vi "RetrieveCustomDiagPacket.vi"(8 "error in":errorcluster, 10 "statusItems":T1[](array[typedef]) {"item code" items=["AccelerationCommand"=6, "AccelerationCommandDrive"=181, "AccelerationCommandRaw"=50, "AccelerationCommandRawCal"=193, "AccelerationError"=223, "AccelerationFeedback"=192, "AccelerationMode"=144, "AccelerationRate"=140, "AccelerationTime"=138, "AccelerationType"=142, "AccuracyCorrectionEndingPosition"=418, "AccuracyCorrectionStartingPosition"=417, "AnalogInput0"=10, "AnalogInput1"=11, "AnalogInput2"=28, "AnalogInput3"=29, "AnalogOutput0"=36, "AnalogOutput1"=37, "AnalogOutput2"=38, "AnalogOutput3"=39, "AutoFocusError"=410, "AxisFault"=49, "AxisParameter"=76, "AxisStatus"=48, "Backlash"=81, "BacklashTarget"=196, "CalibrationAdjustmentState"=416, "CalibrationAdjustmentValue"=200, "CommunicationRealTimeErrors"=93, "CoordinatedDistanceRemaining"=272, "CoordinatedPositionTarget"=46, "CurrentCommand"=8, "CurrentError"=9, "CurrentFeedback"=7, "CurrentFeedbackAverage"=73, "DecelerationMode"=145, "DecelerationRate"=141, "DecelerationTime"=139, "DecelerationType"=143, "DigitalInput"=15, "DigitalOutput"=16, "DistanceLog"=378, "DriveAssert"=453, "DriveCommandsDelayed"=424, "DriveCommandsLost"=425, "DriveCommunicationDelay"=253, "DriveCommunicationDelayLive"=254, "DriveInterfaceCommandCode"=191, "DriveInterfacePacketBit"=261, "DriveInterfacePacketDouble"=189, "DriveInterfacePacketFloat"=190, "DriveInterfacePacketInfoBitValue"=210, "DriveInterfacePacketInt16"=187, "DriveInterfacePacketInt32"=186, "DriveInterfacePacketInt8"=188, "DriveInterfacePacketResponseBit"=262, "DriveInterfacePacketResponseDouble"=259, "DriveInterfacePacketResponseFloat"=260, "DriveInterfacePacketResponseInt16"=257, "DriveInterfacePacketResponseInt32"=256, "DriveInterfacePacketResponseInt8"=258, "DriveInterfacePacketStreamingData"=226, "DriveMotionDelay"=199, "DriveMotionDelayLive"=252, "DriveMotionRate"=198, "DriveSMCMotionState"=168, "DriveStatus"=47, "DriveStatusActual"=99, "FeedforwardCurrent"=208, "FixtureOffset"=18, "FreezeVelocityCommand"=238, "FreezeVelocityFeedback"=239, "GainAffScale"=130, "GainKd1Scale"=333, "GainKiScale"=127, "GainKp1Scale"=334, "GainKpiScale"=129, "GainKposScale"=126, "GainKpScale"=128, "GainVffScale"=131, "GalvoLaserOffDelay"=413, "GalvoLaserOnDelay"=412, "GalvoLaserOutputRaw"=183, "GalvoLaserOutputRawAdvance"=411, "GantryMarkerLatchPosition"=368, "GantryOffset"=91, "GantryRealignState"=100, "HomeState"=82, "InternalPositionOffsets"=241, "JerkCommandRaw"=89, "JogTrajectoryStatus"=116, "MoveReferenceCornerOffset"=359, "MoveReferenceCutterOffset"=358, "MoveReferencePosition"=339, "MoveReferenceTotalOffset"=360, "NormalcyDebug"=84, "PeakCurrent"=78, "PiezoVoltageCommand"=376, "PiezoVoltageFeedback"=377, "PingTest"=117, "PositionCalibration2D"=83, "PositionCalibrationAll"=55, "PositionCalibrationAllDrive"=194, "PositionCommand"=1, "PositionCommandDrive"=98, "PositionCommandPacket"=163, "PositionCommandRaw"=12, "PositionCommandRawBackwardsDiff"=96, "PositionCommandRawCal"=178, "PositionCommandRawUnfiltered"=227, "PositionCommandRollover"=70, "PositionError"=2, "PositionFeedback"=0, "PositionFeedbackAuxiliary"=14, "PositionFeedbackAuxiliaryRollover"=71, "PositionFeedbackDrive"=88, "PositionFeedbackRollover"=69, "PositionOffset"=92, "ProgramPosition"=156, "ProgramPositionCommand"=90, "ProgramPositionFeedback"=107, "ProgramVelocityCommand"=250, "ProgramVelocityFeedback"=251, "SafeZoneState"=323, "ServoRounding"=201, "SpeedTarget"=160, "SpeedTargetActual"=266, "Stability0SettleTime"=86, "Stability1SettleTime"=87, "StatusHighLevelOffsetsLastMsec"=242, "STOStatus"=443, "SuppressedFaults"=225, "TotalMoveTime"=85, "TransformAutoOffset"=101, "TransitionOffsetErrors"=228, "VelocityCommand"=4, "VelocityCommandDrive"=180, "VelocityCommandRaw"=13, "VelocityCommandRawBackwardsDiffDelta"=97, "VelocityCommandRawCal"=179, "VelocityError"=5, "VelocityFeedback"=3, "VelocityFeedbackAverage"=72, "DataCollectionSampleIndex"=161, "DataCollectionSampleTime"=149, "DataCollectionStatus"=255, "DriveModbusMasterInputBits"=354, "DriveModbusMasterInputWords"=352, "DriveModbusMasterOutputBits"=355, "DriveModbusMasterOutputStatusBits"=356, "DriveModbusMasterOutputStatusWords"=357, "DriveModbusMasterOutputWords"=353, "EstimatedProcessorUsage"=236, "FieldbusActiveConnections"=287, "FieldbusConnected"=284, "FieldbusErrorCode"=285, "FieldbusErrorLocation"=286, "FieldbusInactiveConnections"=288, "FieldbusInputs"=340, "FieldbusOutputs"=341, "GlobalVariable"=74, "LibraryCommand"=148, "ModbusMasterInputBits"=344, "ModbusMasterInputWords"=342, "ModbusMasterOutputBits"=345, "ModbusMasterOutputStatusBits"=346, "ModbusMasterOutputStatusWords"=347, "ModbusMasterOutputWords"=343, "ModbusSlaveInputBits"=350, "ModbusSlaveInputWords"=348, "ModbusSlaveOutputBits"=351, "ModbusSlaveOutputWords"=349, "PCModbusMasterConnected"=170, "PCModbusMasterErrorCode"=174, "PCModbusMasterErrorLocation"=176, "PCModbusSlaveConnected"=171, "PCModbusSlaveErrorCode"=175, "PCModbusSlaveErrorLocation"=177, "SafeZoneActiveMask"=321, "SafeZoneViolationMask"=289, "ScopetrigID"=209, "SignalLogState"=270, "StepperVerificationMask"=426, "StopWatchTimer"=197, "SystemParameter"=379, "ThermoCompCompensatingTemperature"=422, "ThermoCompControllingTemperature"=421, "ThermoCompSensorTemperature"=420, "ThermoCompStatus"=423, "Timer"=56, "TimerPerformance"=57, "VirtualBinaryInput"=51, "VirtualBinaryOutput"=52, "VirtualRegisterInput"=53, "VirtualRegisterOutput"=54, "ZYGOPosition1"=164, "ZYGOPosition2"=165, "ZYGOPosition3"=166, "ZYGOPosition4"=167, "ActiveFixtureOffset"=106, "ActiveMoveValid"=435, "AxesSlowdownReason"=448, "CannedFunctionID"=240, "CoordinatedAccelerationCommand"=64, "CoordinatedAccelerationRate"=132, "CoordinatedAccelerationTime"=134, "CoordinatedArcEndAngle"=59, "CoordinatedArcRadius"=60, "CoordinatedArcRadiusError"=61, "CoordinatedArcRadiusReciprocal"=363, "CoordinatedArcStartAngle"=58, "CoordinatedDecelerationRate"=133, "CoordinatedDecelerationTime"=135, "CoordinatedFlags"=45, "CoordinatedGalvoLaserOutput"=169, "CoordinatedMotionRate"=184, "CoordinatedPercentDone"=66, "CoordinatedPositionCommand"=62, "CoordinatedPositionCommandBackwardsDiff"=67, "CoordinatedSpeedCommand"=63, "CoordinatedSpeedTarget"=124, "CoordinatedSpeedTargetActual"=104, "CoordinatedTaskCommand"=185, "CoordinatedTimeScale"=370, "CoordinatedTimeScaleDerivative"=371, "CoordinatedTotalDistance"=65, "CoordinateSystem1I"=118, "CoordinateSystem1J"=119, "CoordinateSystem1K"=120, "CoordinateSystem1Plane"=121, "CriticalSectionActive"=440, "DependentCoordinatedSpeedTarget"=125, "DependentCoordinatedSpeedTargetActual"=105, "EnableAlignmentAxes"=159, "EnableState"=224, "ExecutionMode"=151, "FiberMoveCount"=195, "FiberPower"=273, "FiberPowerOptimal"=274, "FiberPowerSampleCount"=275, "FiberSearchResult"=276, "IFOVAttemptCode"=394, "IFOVCenterPointH"=390, "IFOVCenterPointV"=391, "IFOVCoordinatedAccelerationCommand"=399, "IFOVCoordinatedPositionCommand"=385, "IFOVCoordinatedSpeedCommand"=386, "IFOVFOVDimensionH"=402, "IFOVFOVDimensionV"=403, "IFOVFOVPositionH"=400, "IFOVFOVPositionV"=401, "IFOVGenerationFrameCounter"=382, "IFOVGenerationFrameIndex"=395, "IFOVGenerationTimeModified"=384, "IFOVGenerationTimeOriginal"=383, "IFOVIdealVelocity"=397, "IFOVMaximumVelocity"=396, "IFOVSpeedScale"=380, "IFOVSpeedScaleAverage"=381, "IFOVTrajectoryCount"=392, "IFOVTrajectoryIndex"=393, "ImmediateCommandErrorCode"=329, "ImmediateCommandErrorLocation"=330, "ImmediateState"=155, "LookaheadMovesExamined"=278, "MFO"=123, "MotionBufferElements"=427, "MotionBufferIndex"=432, "MotionBufferIndexLookahead"=433, "MotionBufferMoves"=428, "MotionBufferProcessingBlocked"=434, "MotionBufferRetraceElements"=431, "MotionBufferRetraceMoves"=430, "MotionEngineStage"=367, "MotionLineNumber"=429, "ProfileControlMask"=324, "ProgramLineNumber"=17, "ProgramLineNumberInternal"=322, "ProgramPersistent"=154, "ProgramVariable"=75, "QueueLineCapacity"=326, "QueueLineCount"=325, "QueueStatus"=162, "SchedulerProgramLoopRuns"=438, "SchedulerTaskBlocked"=439, "SchedulerTaskHolds"=437, "Spindle0SpeedTarget"=112, "Spindle1SpeedTarget"=113, "Spindle2SpeedTarget"=114, "Spindle3SpeedTarget"=115, "TaskDoubleVariable"=248, "TaskErrorCode"=79, "TaskErrorLocation"=152, "TaskExecutionLines"=436, "TaskExecutionLinesMaximum"=452, "TaskExecutionTime"=450, "TaskExecutionTimeMaximum"=451, "TaskInfoVariable"=249, "TaskInternalDebug"=398, "TaskMode"=137, "TaskParameter"=77, "TaskReturnVariable"=271, "TaskState"=146, "TaskStateInternal"=147, "TaskStatus0"=108, "TaskStatus1"=109, "TaskStatus2"=110, "TaskWarningCode"=80, "TaskWarningLocation"=153, "ToolNumberActive"=122, "WaitCommandDuration"=103]}, 11 "controller in":refnum<k24>) -> (0 "error out":errorcluster, 1 "data":dbl[](array[numeric]), 3 "controller out":refnum<k24>)   [LabVIEW 2010]
uses:
  c:/aerotech/controller/dev/A3200/pc/labview/2010/bin/Aerotech.A3200.dll
  bin/Aerotech.A3200.dll
  CustomDiagPacketItem.ctl
  c:/aerotech/controller/dev/A3200/pc/labview/2010/bin/Aerotech.A3200.LabVIEW.dll
  bin/Aerotech.A3200.LabVIEW.dll
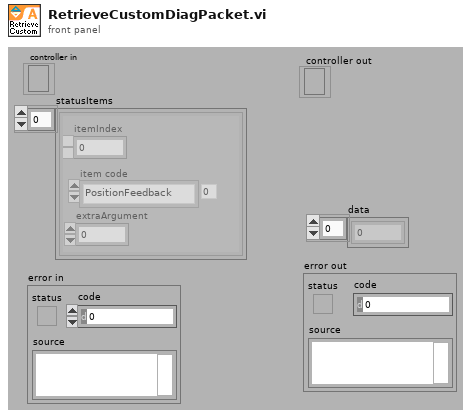
[diagram p1: front panel]
types:
  T1 = typedef "CustomDiagPacketItem.ctl" = cluster{"itemIndex":i16, "item code":u32, "extraArgument":i32}
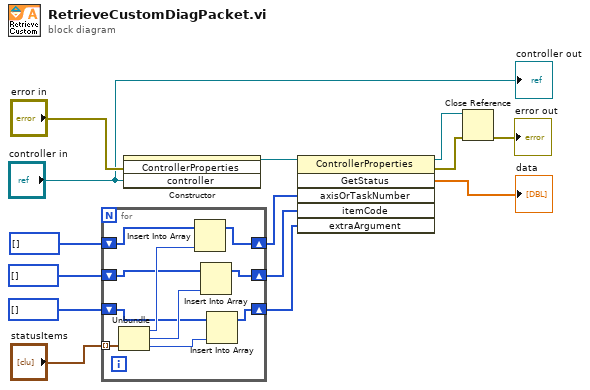
[diagram p0: block diagram]
diagram:
  n1 = for {
    shift-right: [w18] -> w2
    shift-left: i16[] [] ("initialized array") -> [w19]
    shift-right: [w21] -> w3
    shift-left: i16[] [] ("initialized array") -> [w22]
    shift-right: [w15] -> w4
    shift-left: i32[] [] ("initialized array") -> [w17]
    tunnel: "statusItems" -> [w24] mode=indexing
    n2 = Unbundle(w24) -> ("itemIndex"=w23:i16, "item code"=w20:u32, "extraArgument"=w16:i32)
    n3 = Insert Into Array(array=w22, new element=w23) -> (w21:i16[])  [unwired: 1 in]
    n4 = Insert Into Array(array=w19, new element=w20) -> (w18:i16[])  [unwired: 1 in]
    n5 = Insert Into Array(array=w17, new element=w16) -> (w15:i32[])  [unwired: 1 in]
  }
  n6 = constructor class="ControllerProperties"(error in="error in", "controller"="controller in") -> (reference out=w14:refnum<k24>)  [unwired: 2 in, 3 out]
  n7 = invoke class="ControllerProperties" method="GetStatus"(reference=w14, "axisOrTaskNumber"=w3, "itemCode"=w2, "extraArgument"=w4) -> (reference out=w10:refnum<k24>, error out=w11:errorcluster, "GetStatus"=→"data":dbl[])  [unwired: 2 in, 3 out]
  n8 = Close Reference(reference=w10, error in (no error)=w11) -> (error out=→"error out":errorcluster)
  "controller out" <- "controller in"
